vi "Main.vi"(11 "Module Admin":refnum<class "Delacor_lib_QMH_Module Admin.lvclass">) -> ()   [LabVIEW 2019, in "UI.lvlib"]
doc: "This template is based off of the Queued Message Handler design pattern and the Queued Message Handler project template that ships with LabVIEW.\n\nThe main difference is that the queue is private to this module and communication between modules is performed via Broadcast and Request events.\n\nRequest events are wrapped in public API methods and are handled in the Event Handling Loop (EHL) of this VI. Any module can register for Broadcast events sent by this module. The EHL generates messages based on user interface actions.\n\nThe Message Handling Loop (MHL) processes messages generated by the EHL, or by other messages. The messages are string values, so new messages can be added easily to the Message Cases case structure in the MHL. Each message cluster can also provide an optional value for Message Data, which is a variant that can be converted to whatever message-specific data is required.\n_____\nBased on Delacor QMH Project Template 5.0.0.82."
uses:
  UI.lvlib
  <vilib>/Delacor/Delacor QMH/Libraries/Module Admin_class/Delacor_lib_QMH_Module Admin.lvclass
  Module Data--cluster.ctl
  Stop Argument--cluster.ctl
  <vilib>/Delacor/Delacor QMH/Libraries/Message Queue_class/Delacor_lib_QMH_Message Queue.lvclass/Delacor_lib_QMH_Message Queue.ctl
  <vilib>/Delacor/Delacor QMH/Libraries/Module Admin_class/Delacor_lib_QMH_Module Admin.lvclass/Delacor_lib_QMH_Module Admin.ctl
  <vilib>/Utility/miscctls.llb/LVPointTypeDef.ctl
  <vilib>/Delacor/Delacor QMH/Libraries/Message Queue_class/Delacor_lib_QMH_Enqueue Message (Single).vi
  <vilib>/Delacor/Delacor QMH/Libraries/Module Admin_class/Delacor_lib_QMH_Get External Launch.vi
  <vilib>/Utility/error.llb/Error Cluster From Error Code.vi
  <vilib>/ErrorRing/Error Ring.xnode
  <vilib>/Delacor/Delacor QMH/Libraries/Message Queue_class/Delacor_lib_QMH_Message Queue.lvclass
  Acquisition HL/Acquisition HL.lvlib
panel:
  in  "Stop Acq":bool
  in  "Start Acq":bool
  out "error out":errorcluster
  out "Status":string
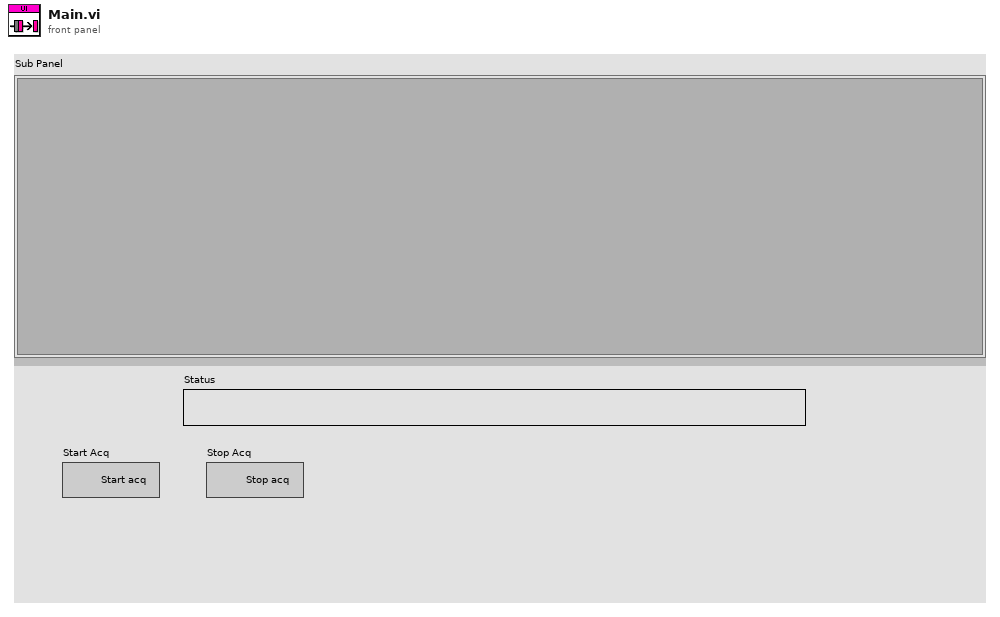
[diagram p1: front panel]
types:
  T1 = typedef "UI.lvlib/Request Events--cluster.ctl" = cluster{"Stop Module":refnum<user-event>, "Show Panel":refnum<user-event>, "Hide Panel":refnum<user-event>, "Get Module Execution Status":refnum<user-event>, "Show Diagram":refnum<user-event>}
  T2 = typedef "Acquisition HL.lvlib/Broadcast Events--cluster.ctl" = cluster{"Module Did Init":refnum<user-event>, "Status Updated":refnum<user-event>, "Error Reported":refnum<user-event>, "Module Did Stop":refnum<user-event>, "Update Module Execution Status":refnum<user-event>}
  T3 = typedef "UI.lvlib/Module Data--cluster.ctl" = cluster{"Status":string}
  T4 = enum32{"invalid lock state", "Not Locked", "Locked (No Password)", "Password-protected"}
  T5 = typedef "UI.lvlib/Stop Argument--cluster.ctl" = cluster{"Origin":string, "Exit via Stop Module Req?":bool, "Wait for Module to stop?":bool}
  T6 = enum32{"Invalid", "Standard", "Closed", "Hidden", "Minimized", "Maximized"}
  T7 = typedef "LVPointTypeDef.ctl" = cluster{"Horizontal":i16, "Vertical":i16}
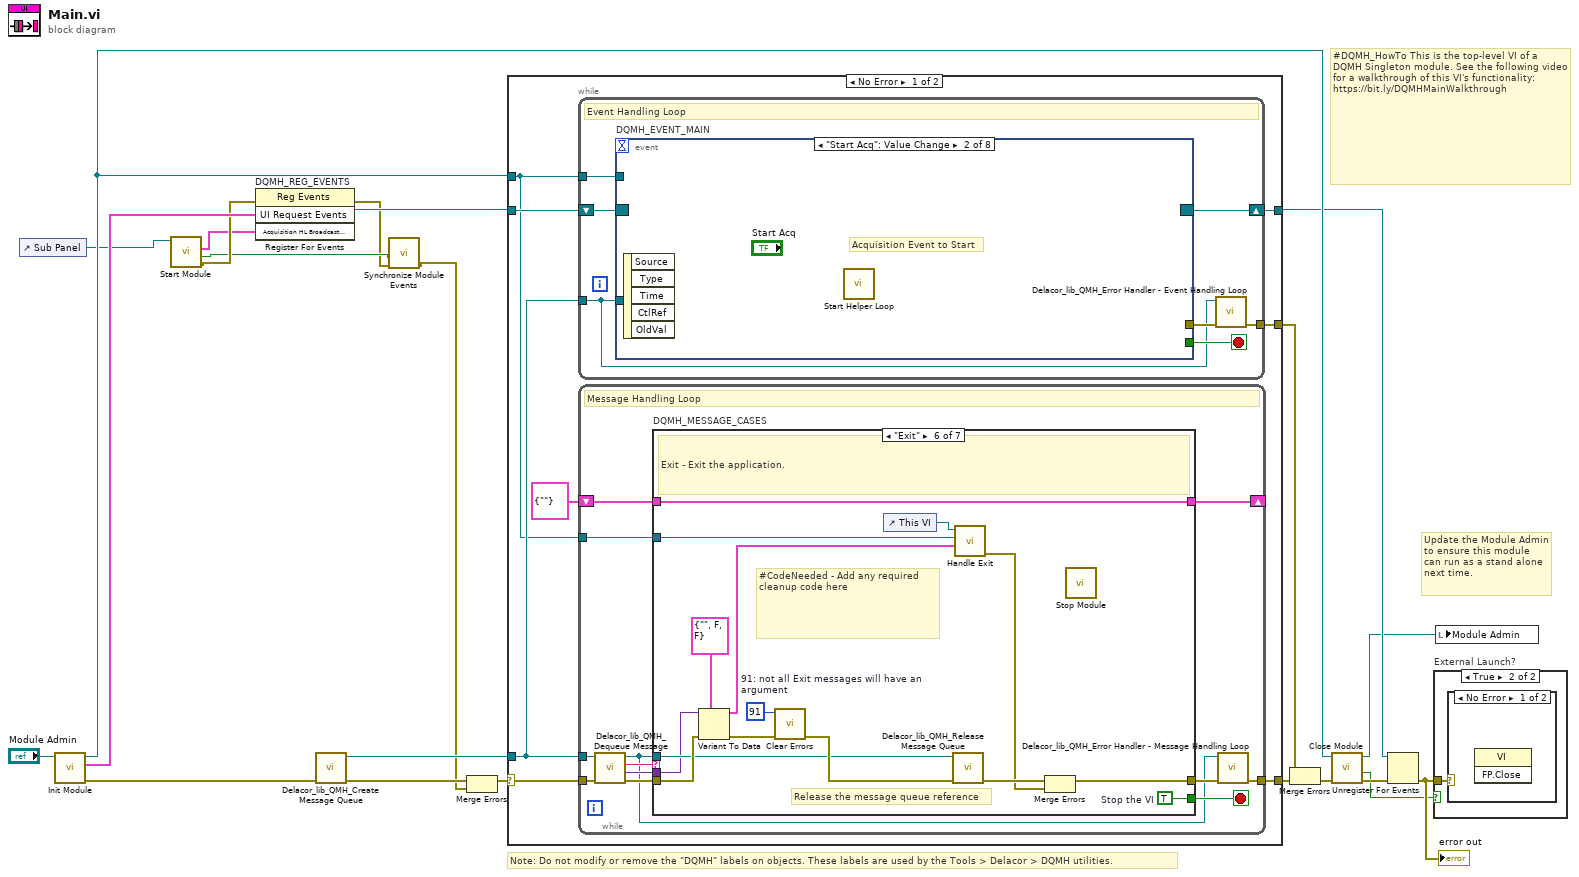
[diagram p0: block diagram]
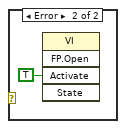
[diagram p3: hidden frame]
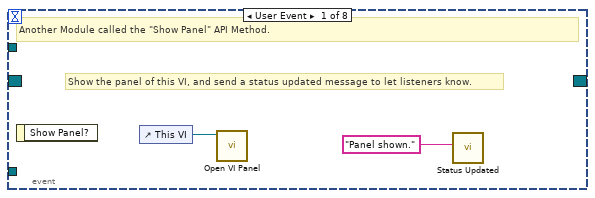
[diagram p4: hidden frame]
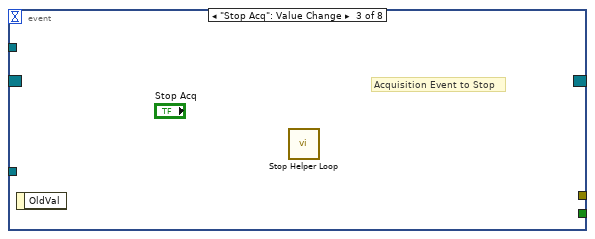
[diagram p5: hidden frame]
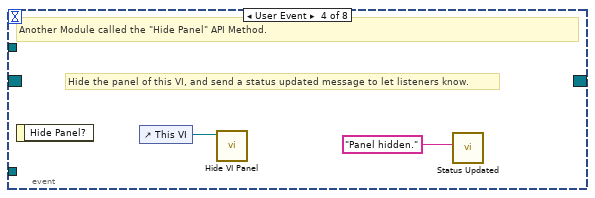
[diagram p6: hidden frame]
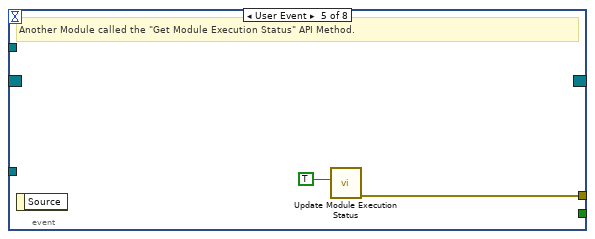
[diagram p7: hidden frame]
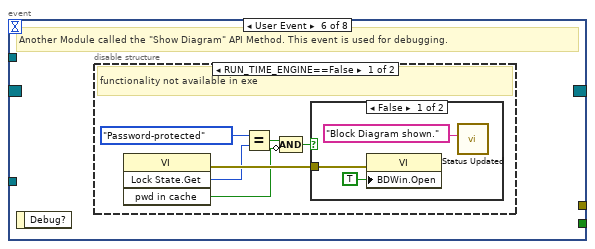
[diagram p8: hidden frame]
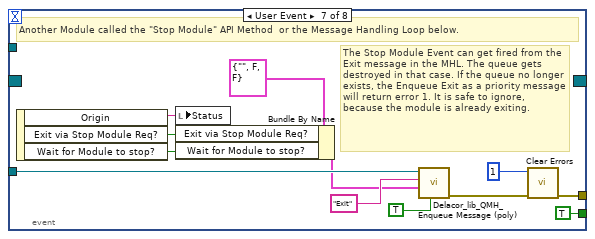
[diagram p11: hidden frame]
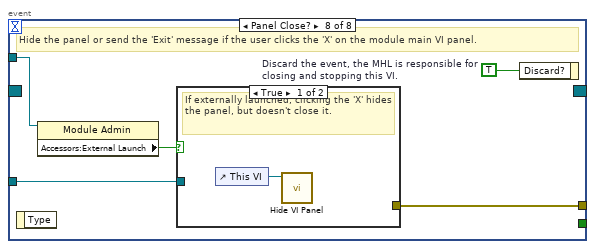
[diagram p12: hidden frame]
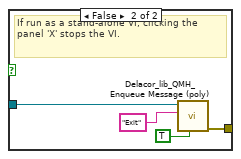
[diagram p13: hidden frame]
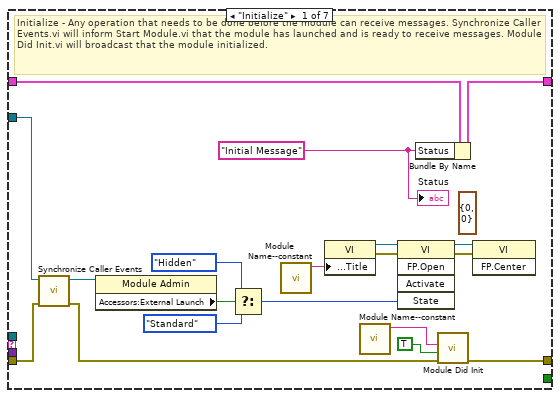
[diagram p14: hidden frame]
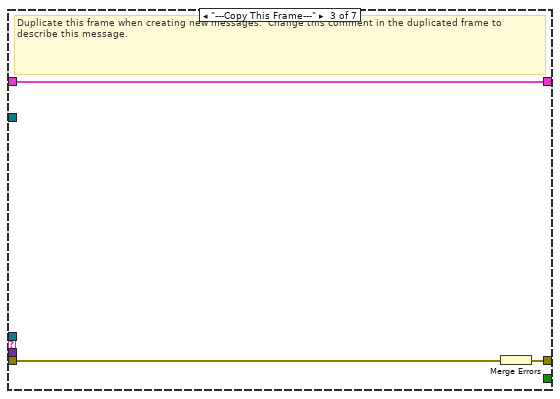
[diagram p16: hidden frame]
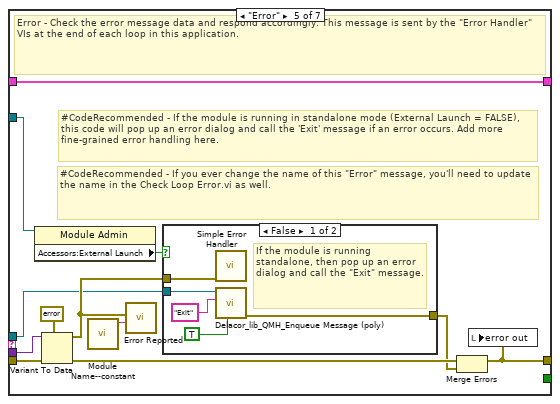
[diagram p18: hidden frame]
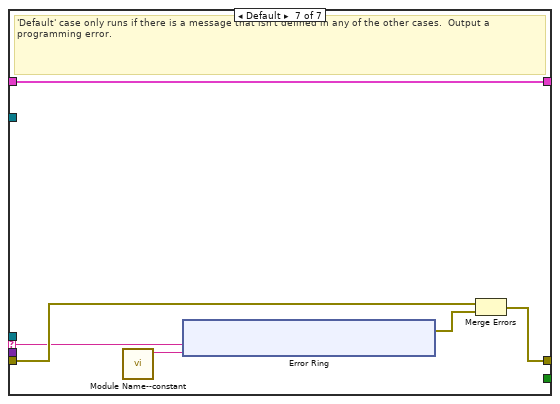
[diagram p20: hidden frame]
diagram:
  # "#DQMH_HowTo This is the top-level VI of a DQMH Singleton module. See the following video for a walkthrough of this VI's functionality: https://bit.ly/DQMHMainWalkthrough"
  # "Note: Do not modify or remove the \"DQMH\" labels on objects. These labels are used by the Tools > Delacor > DQMH utilities."
  # "Update the Module Admin to ensure this module can run as a stand alone next time."
  n1 = control-ref of="Sub Panel"() -> (w1:refnum<vi>)
  n2 = call "Init Module.vi"("Singleton Module Admin in"="Module Admin") -> ("error out"=w21:errorcluster, "UI Request Events"=w11:T1, "Singleton Module Admin out"=w14:refnum<class "Delacor_lib_QMH_Module Admin.lvclass">)  [unwired: 8 in]
  n3 = call "Start Module.vi"("ACQ HL Panel"=w1) -> ("error out"=w6:errorcluster, "Wait for Event Sync?"=w4:bool, "Acquisition HL Broadcast Events"=w5:T2)  [unwired: 7 in, 1 out]
  n4 = register-events "DQMH_REG_EVENTS"(error in=w6, w11, w5) -> (reference out=w12:refnum<event-registration>, error out=w3:errorcluster)  [unwired: 1 in]
  n5 = call <vilib>:"Delacor_lib_QMH_Create Message Queue.vi"("error in (no error)"=w21) -> ("error out"=w16:errorcluster, "Message Queue"=w10:refnum<class "Delacor_lib_QMH_Message Queue.lvclass">)  [unwired: 9 in]
  n6 = call "Synchronize Module Events.vi"("error in (no error)"=w3, "Wait for Event Sync?"=w4) -> ("error out"=w2:errorcluster)  [unwired: 9 in]
  n7 = Merge Errors(w16, w2) -> (w15:errorcluster)
  n8 = case shown="No Error" w15 {
    selector: w15 -> [w28 w161]
    tunnel: [w30 w160] -> w22
    tunnel: [w27 w166] -> w13
    tunnel: w12 -> [w25 w166]
    tunnel: w10 -> [w24 w159]
    tunnel: [w29 _] -> w19
    tunnel: w14 -> [w23 w162]
    frame No Error {
      n9 = while {
        tunnel: w24 -> [w31]
        shift-right: [w34] -> w27
        shift-left: w25 -> [w35]
        tunnel: [w36] -> w29
        tunnel: w23 -> [w32]
        stop <- w33 stop-if-true
        # "Event Handling Loop"
        n10 = event "DQMH_EVENT_MAIN" shown="[1] \"Start Acq\": Value Change" {
          selector: w35 -> [_ _ _ _ _ _ _ _]
          dyn-events: [_ _ _ _ _ _ _ _] -> w34
          timeout: _ -> [_ _ _ _ _ _ _ _]
          tunnel: [_ _ _ _ _ _ TRUE ("Discard?") _] -> w33
          tunnel: w31 -> [_ _ _ _ _ _ w60 w67]
          tunnel: [_ _ _ _ w43 _ w63 w69] -> w37
          tunnel: w32 -> [_ _ _ _ _ _ _ w66]
          event User Event {
            # "Show the panel of this VI, and send a status updated message to let listeners know."
            # "Another Module called the \"Show Panel\" API Method."
            n11 = event-data() -> ()  [unwired: 1 in, 1 out]
            n12 = control-ref of="This VI"() -> (w39:refnum<vi>)
            n13 = call "Open VI Panel.vi"("VI"=w39) -> ()  [unwired: 10 in, 1 out]
            n14 = call "Status Updated.vi"("Status"="Panel shown." ("format string")) -> ()  [unwired: 10 in, 1 out]
          }
          event "Start Acq": Value Change {
            # "Acquisition Event to Start"
            n15 = event-data() -> ()  [unwired: 1 in, 5 out]
            n16 = call "Start Helper Loop.vi"() -> ()  [unwired: 11 in, 1 out]
          }
          event "Stop Acq": Value Change {
            # "Acquisition Event to Stop"
            n17 = event-data() -> ()  [unwired: 1 in, 1 out]
            n18 = call "Stop Helper Loop.vi"() -> ()  [unwired: 11 in, 1 out]
          }
          event User Event {
            # "Hide the panel of this VI, and send a status updated message to let listeners know."
            # "Another Module called the \"Hide Panel\" API Method."
            n19 = event-data() -> ()  [unwired: 1 in, 1 out]
            n20 = control-ref of="This VI"() -> (w41:refnum<vi>)
            n21 = call "Hide VI Panel.vi"("VI"=w41) -> ()  [unwired: 10 in, 1 out]
            n22 = call "Status Updated.vi"("Status"="Panel hidden." ("format string")) -> ()  [unwired: 10 in, 1 out]
          }
          event User Event {
            # "Another Module called the \"Get Module Execution Status\" API Method."
            n23 = event-data() -> ()  [unwired: 1 in, 1 out]
            n24 = call "Update Module Execution Status.vi"("Running?"=TRUE) -> ("error out"=w43:errorcluster)  [unwired: 10 in]
          }
          event User Event {
            # "Another Module called the \"Show Diagram\" API Method. This event is used for debugging."
            n25 = event-data() -> ()  [unwired: 1 in, 1 out]
            n26 = disable-structure shown="RUN_TIME_ENGINE==False" {
              frame condition #0 (active) {
                # "functionality not available in exe"
                n27 = invoke class="VI" method="Lock State.Get"() -> (error out=w49:errorcluster, "Get Lock State"=w48:T4, "pwd in cache"=w45:bool)  [unwired: 4 in, 1 out]
                n28 = Equal?(x=T4."Password-protected", y=w48) -> (x = y?=w46:bool)
                n29 = Compound Arithmetic op=AND(w46, invert w45) -> (w44:bool)
                n30 = case shown="False" w44 {
                  tunnel: w49 -> [w52 _]
                  frame False {
                    n31 = property class="VI"(error in=w52, "BDWin.Open"=TRUE ("Block Diagram Window:Open")) -> ()  [unwired: 1 in, 2 out]
                    n32 = call "Status Updated.vi"("Status"="Block Diagram shown." ("format string")) -> ()  [unwired: 10 in, 1 out]
                  }
                  frame True {
                    # "Password-protected VI, and the password is not in the cache. Do not show the diagram."
                  }
                }
              }
              frame condition #1 {
              }
            }
          }
          event User Event {
            # "The Stop Module Event can get fired from the Exit message in the MHL. The queue gets destroyed in that case. If the queue no longer exists, the Enqueue Exit as a priority message will return error 1. It is safe to ignore, because the module is already exiting."
            # "Another Module called the \"Stop Module\" API Method  or the Message Handling Loop below."
            n33 = event-data() -> ("Origin"=w59:string, "Exit via Stop Module Req?"=w55:bool, "Wait for Module to stop?"=w54:bool)  [unwired: 1 in]
            n34 = local write "Status"(w59) -> ()
            n35 = Bundle By Name(cluster=T5 {"Origin"="", "Exit via Stop Module Req?"=FALSE, "Wait for Module to stop?"=FALSE} ("Stop Argument"), "Exit via Stop Module Req?"=w55, "Wait for Module to stop?"=w54) -> (w53:T5)
            n36 = call-poly <vilib>:"Delacor_lib_QMH_Enqueue Message (poly).vi"("Priority Message? (F)"=TRUE, "Message Data"=w53, "Message"="Exit", "Message Queue in"=w60) -> ("error out"=w64:errorcluster)  [unwired: 6 in, 1 out]
            n37 = call <vilib>:"Clear Errors.vi"("error in (no error)"=w64, "specific error code to clear (0: all)"=1) -> ("error out"=w63:errorcluster)  [unwired: 4 in, 1 out]
          }
          event Panel Close? {
            w68 = TRUE  # Discard the event, the MHL is responsible for closing and stopping this VI.
            # "Hide the panel or send the 'Exit' message if the user clicks the 'X' on the module main VI panel."
            n38 = event-data() -> ()  [unwired: 1 in, 1 out]
            n39 = property class="Module Admin"(reference=w66) -> ("Accessors:External Launch"=w65:bool)  [unwired: 1 in, 2 out]
            n40 = case shown="True" w65 {
              tunnel: w67 -> [_ w73]
              tunnel: [_ w74] -> w69
              frame True {
                # "If externally launched, clicking the 'X' hides the panel, but doesn't close it."
                n41 = control-ref of="This VI"() -> (w70:refnum<vi>)
                n42 = call "Hide VI Panel.vi"("VI"=w70) -> ()  [unwired: 10 in, 1 out]
              }
              frame False {
                # "If run as a stand-alone VI, clicking the panel 'X' stops the VI."
                n43 = call-poly <vilib>:"Delacor_lib_QMH_Enqueue Message (poly).vi"("Priority Message? (F)"=TRUE, "Message"="Exit", "Message Queue in"=w73) -> ("error out"=w74:errorcluster)  [unwired: 7 in, 1 out]
              }
            }
            n44 = event-data("Discard?"=w68) -> ()  [unwired: 1 in, 1 out]
          }
        }
        n45 = call-dynamic "Delacor_lib_QMH_Error Handler - Event Handling Loop.vi"("error in (no error)"=w37, "Message Queue in"=w31) -> ("dup error in"=w36:errorcluster)  [unwired: 8 in, 1 out]
      }
      n46 = while {
        tunnel: w24 -> [w77]
        shift-right: [w81] -> _
        shift-left: T3 {"Status"=""} ("Data Cluster") -> [w82]
        tunnel: w28 -> [w85]
        tunnel: [w83] -> w30
        tunnel: w23 -> [w75]
        stop <- w80 stop-if-true
        # "Message Handling Loop"
        n47 = call-dynamic "Delacor_lib_QMH_Dequeue Message.vi"("error in (no error)"=w85, "Message Queue in"=w77) -> ("error out"=w84:errorcluster, "Message Data"=w78:variant, "Message"=w79:string, "Message Queue out"=w76:refnum<class "Delacor_lib_QMH_Message Queue.lvclass">)  [unwired: 6 in]
        n48 = case "DQMH_MESSAGE_CASES" shown="\"Exit\"" w79 {
          selector: w79 -> [_ _ _ _ _ _ w146]
          tunnel: w76 -> [_ _ _ _ w116 w138 _]
          tunnel: w84 -> [w103 w107 w110 w112 w123 w144 w148]
          tunnel: [w101 w107 w109 w112 w119 w141 w149] -> w86
          tunnel: w82 -> [w92 w106 w108 w111 w118 w137 w147]
          tunnel: [w91 w106 w108 w111 w118 w137 w147] -> w81
          tunnel: [_ _ _ _ _ w136 _] -> w80
          tunnel: w78 -> [_ _ _ _ w117 w135 _]
          tunnel: w75 -> [w93 _ _ _ w115 w130 _]
          frame "Initialize" {
            (unwired) T7 {"Horizontal"=0, "Vertical"=0} ("Origin")
            w87 = "Initial Message" ("Initial Message")
            # "Initialize - Any operation that needs to be done before the module can receive messages. Synchronize Caller Events.vi will inform Start Module.vi that the module has launched and is ready to receive messages. Module Did Init.vi will broadcast that the module initialized."
            n49 = call "Synchronize Caller Events.vi"("error in (no error)"=w103, "Singleton Module Admin in"=w93) -> ("error out"=w102:errorcluster, "Singleton Module Admin out"=w88:refnum<class "Delacor_lib_QMH_Module Admin.lvclass">)  [unwired: 8 in]
            n50 = property class="Module Admin"(reference=w88) -> ("Accessors:External Launch"=w97:bool)  [unwired: 1 in, 2 out]
            n51 = Select(t=T6."Hidden" ("State"), s=w97, f=T6."Standard" ("State")) -> (s? t:f=w94:T6)
            n52 = call "Module Name--constant.vi"() -> ("Module Name"=w100:string)  [unwired: 11 in]
            n53 = property class="VI"("Front Panel.Title"=w100) -> (reference out=w99:refnum<vi>, error out=w105:errorcluster)  [unwired: 2 in]
            n54 = call "Module Name--constant.vi"() -> ("Module Name"=w89:string)  [unwired: 11 in]
            n55 = invoke class="VI" method="FP.Open"(reference=w99, error in=w105, "State"=w94) -> (reference out=w98:refnum<vi>, error out=w104:errorcluster)  [unwired: 2 in, 3 out]
            n56 = Bundle By Name(cluster=w92, "Status"=w87) -> (w91:T3)
            n57 = call "Module Did Init.vi"("error in (no error)"=w102, "Initialized?"=TRUE, "Origin"=w89) -> ("error out"=w101:errorcluster)  [unwired: 8 in]
            n58 = invoke class="VI" method="FP.Center"(reference=w98, error in=w104) -> ()  [unwired: 1 in, 3 out]
            "Status" <- w87
          }
          frame "--- Module Specific ---" {
            # "Separator -- The following cases handle messages specific to this Module."
          }
          frame "---Copy This Frame---" {
            # "Duplicate this frame when creating new messages.  Change this comment in the duplicated frame to describe this message."
            n59 = Merge Errors(w110) -> (w109:errorcluster)
          }
          frame "--- Exit and Error Handling---" {
            # "Separator - The following cases handle errors and exit messages."
          }
          frame "Error" {
            # "#CodeRecommended - If you ever change the name of this \"Error\" message, you'll need to update the name in the Check Loop Error.vi as well."
            # "#CodeRecommended - If the module is running in standalone mode (External Launch = FALSE), this code will pop up an error dialog and call the 'Exit' message if an error occurs. Add more fine-grained error handling here."
            # "Error - Check the error message data and respond accordingly. This message is sent by the \"Error Handler\" VIs at the end of each loop in this application."
            n60 = property class="Module Admin"(reference=w115) -> ("Accessors:External Launch"=w114:bool)  [unwired: 1 in, 2 out]
            n61 = Variant To Data(error in=w123, type=errorcluster {"status"=FALSE, "code"=0, "source"=""} ("error constant"), Variant=w117) -> (data=w124:errorcluster, error out=w121:errorcluster)
            n62 = call "Module Name--constant.vi"() -> ("Module Name"=w113:string)  [unwired: 11 in]
            n63 = call "Error Reported.vi"("Additional Information"=w113, "Error"=w124) -> ()  [unwired: 9 in, 1 out]
            n64 = case shown="False" w114 {
              tunnel: [w129 _] -> w120
              tunnel: w116 -> [w127 _]
              tunnel: w124 -> [w128 _]
              frame False {
                # "If the module is running standalone, then pop up an error dialog and call the \"Exit\" message."
                n65 = call <vilib>:"Simple Error Handler.vi"("error in (no error)"=w128) -> ()  [unwired: 4 in, 5 out]
                n66 = call-poly <vilib>:"Delacor_lib_QMH_Enqueue Message (poly).vi"("Priority Message? (F)"=TRUE, "Message"="Exit", "Message Queue in"=w127) -> ("error out"=w129:errorcluster)  [unwired: 7 in, 1 out]
              }
              frame True {
                # "If the module was launched externally, calling the Error Reported broadcast VI is the only action performed by the \"Error\" message. The module's caller can then process the error appropriately."
              }
            }
            n67 = Merge Errors(w121, w120) -> (w119:errorcluster)
            n68 = local write "error out"(w119) -> ()
          }
          frame "Exit" {
            w134 = 91  # 91: not all Exit messages will have an argument
            w136 = TRUE  # Stop the VI
            # "Release the message queue reference"
            # "#CodeNeeded - Add any required cleanup code here"
            # "Exit - Exit the application."
            n69 = Variant To Data(error in=w144, type=T5 {"Origin"="", "Exit via Stop Module Req?"=FALSE, "Wait for Module to stop?"=FALSE} ("Stop Argument"), Variant=w135) -> (data=w132:T5, error out=w140:errorcluster)
            n70 = call <vilib>:"Clear Errors.vi"("error in (no error)"=w140, "specific error code to clear (0: all)"=w134) -> ("error out"=w143:errorcluster)  [unwired: 4 in, 1 out]
            n71 = control-ref of="This VI"() -> (w131:refnum<vi>)
            n72 = call-dynamic "Delacor_lib_QMH_Release Message Queue.vi"("error in (no error)"=w143, "Message Queue"=w138) -> ("error out"=w142:errorcluster)  [unwired: 9 in]
            n73 = call "Handle Exit.vi"("Stop Argument"=w132, "Admin in"=w130, "VI reference"=w131) -> ("error out"=w139:errorcluster)  [unwired: 7 in, 1 out]
            n74 = Merge Errors(w142, w139) -> (w141:errorcluster)
            n75 = call "Stop Module.vi"() -> ()  [unwired: 11 in, 1 out]
          }
          frame Default {
            # "'Default' case only runs if there is a message that isn't defined in any of the other cases.  Output a programming error."
            n76 = call "Module Name--constant.vi"() -> ("Module Name"=w145:string)  [unwired: 11 in]
            n77 = xnode "Error Ring"("parameter 0"=w146, "parameter 1"=w145) -> ("error out"=w150:errorcluster)
            n78 = Merge Errors(w148, w150) -> (w149:errorcluster)
          }
        }
        n79 = call-dynamic "Delacor_lib_QMH_Error Handler - Message Handling Loop.vi"("error in (no error)"=w86, "Message Queue in"=w76) -> ("dup error in"=w83:errorcluster)  [unwired: 8 in, 1 out]
      }
    }
    frame Error {
      # "Synchronize Caller Events.vi will inform Start Module.vi that the module has launched and will let the code calling Start Module.vi register for broadcasts and would permit the caller receive the broadcast that an error occurred at launch time."
      n80 = call-dynamic "Delacor_lib_QMH_Release Message Queue.vi"("error in (no error)"=w161, "Message Queue"=w159) -> ("error out"=w160:errorcluster)  [unwired: 9 in]
      n81 = call "Synchronize Caller Events.vi"("Singleton Module Admin in"=w162) -> ("error out"=w167:errorcluster)  [unwired: 9 in, 1 out]
      n82 = call "Module Name--constant.vi"() -> ("Module Name"=w165:string)  [unwired: 11 in]
      n83 = Format Into String(format string="An error occurred during initialization. %s is no longer running.", w165) -> (resulting string=w163:string)  [unwired: 2 in, 1 out]
      n84 = Merge Errors(w160, w167) -> (w168:errorcluster)
      n85 = call "Error Reported.vi"("Additional Information"=w163, "Error"=w168) -> ()  [unwired: 9 in, 1 out]
    }
  }
  n86 = Merge Errors(w19, w22) -> (w18:errorcluster)
  n87 = call "Close Module.vi"("error in (no error)"=w18, "Module Admin in"=w14) -> ("error out"=w20:errorcluster, "External Launch"=w7:bool, "Module Admin out"=w8:refnum<class "Delacor_lib_QMH_Module Admin.lvclass">)  [unwired: 7 in]
  n88 = Unregister For Events(event registration refnum=w13, error in=w20) -> (error out=w17:errorcluster)
  "error out" <- w17
  n89 = case "External Launch?" shown="True" w7 {
    tunnel: w17 -> [_ w169]
    frame False {
    }
    frame True {
      n90 = case shown="No Error" w169 {
        frame No Error {
          n91 = invoke class="VI" method="FP.Close"() -> ()  [unwired: 3 in, 3 out]
        }
        frame Error {
          n92 = invoke class="VI" method="FP.Open"("Activate"=TRUE ("Activate?")) -> ()  [unwired: 4 in, 5 out]
        }
      }
    }
  }
  n93 = local write "Module Admin"(w8) -> ()
